vi "balloon入队列.vi"(10 "报警内容":cluster{"报警内容":string, "报警分析":string}, 11 "队列":refnum<queue>) -> (3 "队列输出":refnum<queue>)   [LabVIEW 2016, in "斯坦道CODcr.lvlib"]
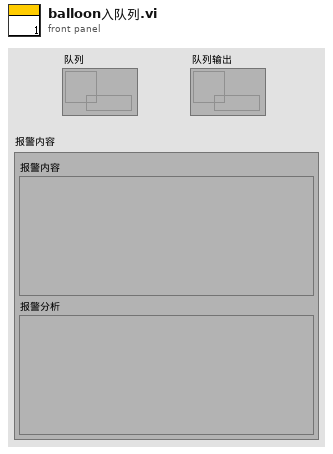
[diagram p1: front panel]
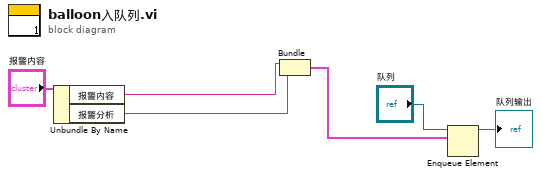
[diagram p0: block diagram]
diagram:
  n1 = Unbundle By Name("报警内容") -> ("报警内容"=w2:string, "报警分析"=w1:string)
  n2 = Bundle("报警内容"=w2, "报警分析"=w1) -> (w6:cluster{"报警内容":string, "报警分析":string})  [unwired: 1 in]
  n3 = Enqueue Element(queue="队列", element=w6) -> (queue out=→"队列输出":refnum<queue>)  [unwired: 2 in, 2 out]
